vi "Measure One Point.vi"(8 "error in (no error)":errorcluster, 11 "DMM in":refnum<class "DMM.lvclass">) -> (0 "error out":errorcluster, 3 "DMM out":refnum<class "DMM.lvclass">)   [LabVIEW 2020, in "DMM.lvclass"]
uses:
  DMM.lvclass
  DMM.lvclass/DMM.ctl
  <vilib>/numeric/Random Number (Range) DBL.vi
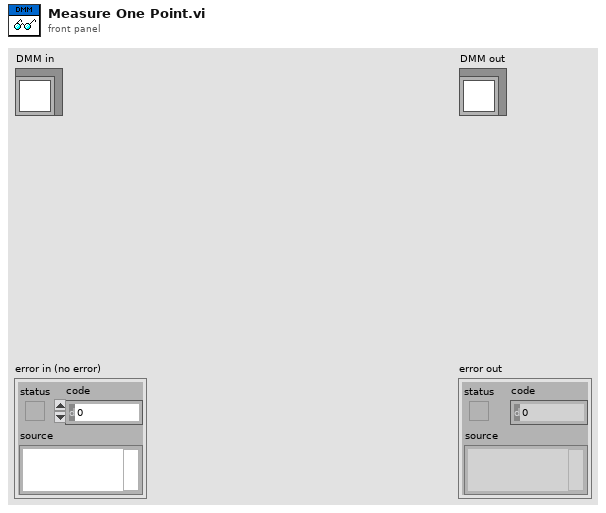
[diagram p1: front panel]
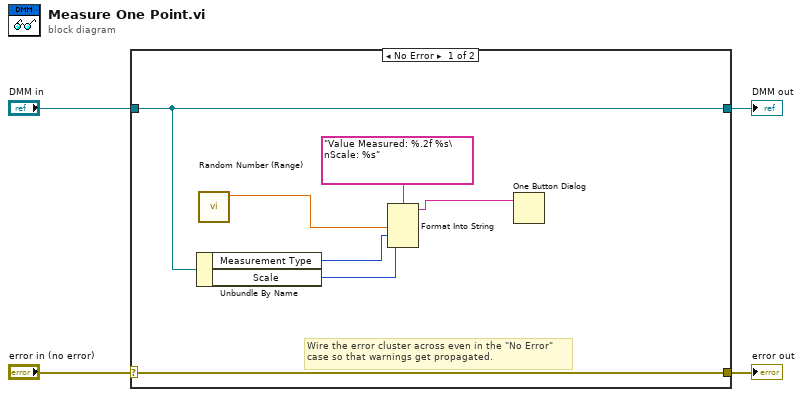
[diagram p0: block diagram]
diagram:
  n1 = case shown="No Error" "error in (no error)" {
    selector: "error in (no error)" -> [w11 w13]
    tunnel: [w11 w13] -> w3
    tunnel: [w10 w12] -> w1
    tunnel: "DMM in" -> [w10 w12]
    frame No Error {
      # "Wire the error cluster across even in the \"No Error\"\ncase so that warnings get propagated."
      n2 = Unbundle By Name(w10) -> ("Measurement Type"=w7:enum16{"DCV", "ACV", "DCI", "ACI"}, "Scale"=w6:enum16{"1u", "1m", "1", "10", "100", "1k", "1M"})
      n3 = call-poly <vilib>:"Random Number (Range).vi"() -> ("number"=w8:dbl)  [unwired: 11 in]
      n4 = Format Into String(format string="Value Measured: %.2f %s\nScale: %s", w8, w7, w6) -> (resulting string=w5:string)  [unwired: 2 in, 1 out]
      n5 = One Button Dialog(message=w5) -> ()  [unwired: 1 in, 1 out]
    }
    frame Error {
    }
  }
  "error out" <- w3
  "DMM out" <- w1
